vi "Initialize.vi"(8 "error in":errorcluster, 11 "Plugin in":refnum<class "RPM Plugin.lvclass">) -> (0 "error out":errorcluster, 3 "Plugin out":refnum<class "RPM Plugin.lvclass">)   [LabVIEW 2020, in "RPM Plugin.lvlib" / "RPM Plugin.lvclass"]
uses:
  RPM Plugin.lvclass
  C:/Program Files/National Instruments/LabVIEW 2020/vi.lib/FlexLogger/SDK/PluginSDK.lvlibp/PEFClasses/SDK/Plugin/Plugin.lvclass
  <vilib>/FlexLogger/SDK/PluginSDK.lvlibp/PEFClasses/SDK/Processing Element/Timing Parameters.ctl
  <vilib>/FlexLogger/SDK/PluginSDK.lvlibp/PEFClasses/SDK/Processing Element/Timing Method.ctl
  <vilib>/FlexLogger/SDK/PluginSDK.lvlibp/PEFClasses/SDK/Producer Channel/Producer Channel.lvclass
  C:/Program Files/National Instruments/LabVIEW 2020/vi.lib/FlexLogger/SDK/PluginSDK.lvlibp/PEFClasses/SDK/Channel/Channel.lvclass
  <vilib>/FlexLogger/SDK/PluginSDK.lvlibp/PEFClasses/SDK/Plugin/ParameterAccess/Write String.vi
  <vilib>/FlexLogger/SDK/PluginSDK.lvlibp/PEFClasses/SDK/Plugin/ParameterAccess/Write DBL.vi
  <vilib>/FlexLogger/SDK/PluginSDK.lvlibp/PEFClasses/SDK/Producer Channel/Create Producer Channel.vi
  <vilib>/FlexLogger/SDK/PluginSDK.lvlibp/PEFClasses/SDK/Channel/ParameterAccess/Write DBL.vi
  <vilib>/FlexLogger/SDK/PluginSDK.lvlibp/PEFClasses/SDK/Plugin/Plugin.lvclass
  <vilib>/FlexLogger/SDK/PluginSDK.lvlibp/PEFClasses/SDK/Channel/Channel.lvclass
  <vilib>/FlexLogger/SDK/PluginSDK.lvlibp
  <vilib>/FlexLogger/SDK/PluginSDK.lvlibp/PEFClasses/SDK/Processing Element/Processing Element.lvclass
  C:/Program Files/National Instruments/LabVIEW 2020/vi.lib/FlexLogger/SDK/PluginSDK.lvlibp/PEFClasses/SDK/Processing Element/Processing Element.lvclass
  D:/AE/Transportation/Schwing Stetter/RPM Plugin/RPM Plugin/RPM Plugin.lvclass
  C:/Program Files/National Instruments/LabVIEW 2020/vi.lib/FlexLogger/SDK/PluginSDK.lvlibp/PEFClasses/SDK/Producer Channel/Producer Channel.lvclass
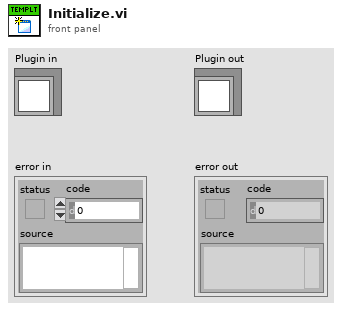
[diagram p1: front panel]
types:
  T1 = typedef "PluginSDK.lvlibp/Processing Element.lvclass/Timing Parameters.ctl" = cluster{"Timing Method":T2, "Timing Period (ms)":i32}
  T2 = typedef "PluginSDK.lvlibp/Processing Element.lvclass/Timing Method.ctl" = enum16{"Periodic", "Immediate", "On Data Ready", "Triggered"}
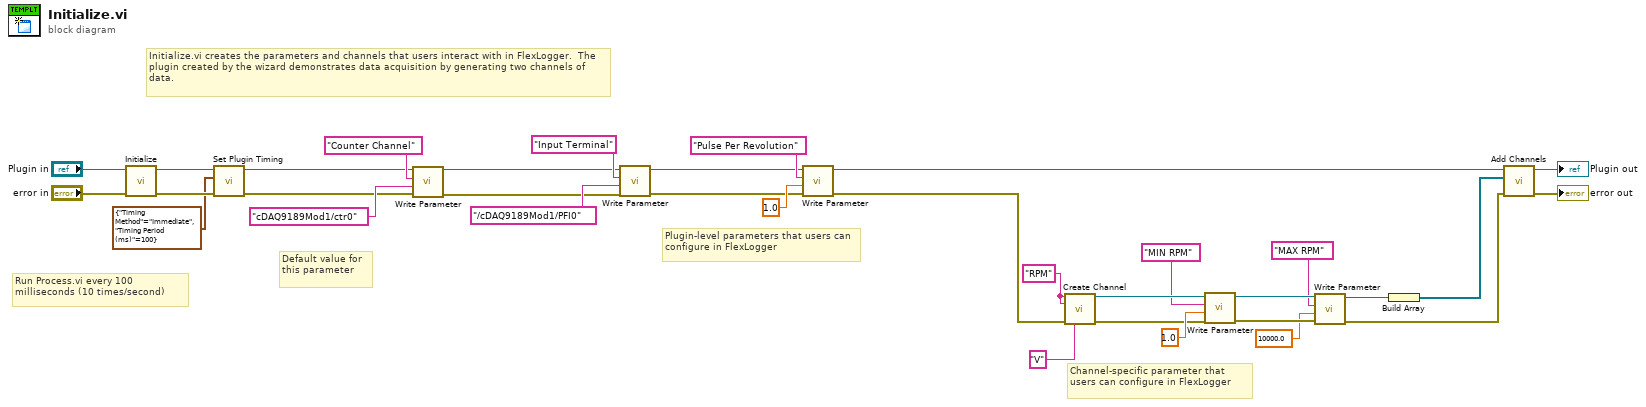
[diagram p0: block diagram]
diagram:
  w8 = "RPM" ("Unique Channel Identifier")
  # "Channel-specific parameter that users can configure in FlexLogger"
  # "Default value for this parameter"
  # "Plugin-level parameters that users can configure in FlexLogger"
  # "Run Process.vi every 100 milliseconds (10 times/second)"
  # "Initialize.vi creates the parameters and channels that users interact with in FlexLogger.  The plugin created by the wizard demonstrates data acquisition by generating two channels of data."
  n1 = call-parent "Initialize.vi"("error in (no error)"="error in", "Plugin in"="Plugin in") -> ("error out"=w24:errorcluster, "Plugin out"=w22:refnum<class "RPM Plugin.lvclass">)  [unwired: 8 in]
  n2 = call <vilib>:"Set Plugin Timing.vi"("error in (no error)"=w24, "Timing Parameters"=T1 {"Timing Method"=enum."Immediate", "Timing Period (ms)"=100}, "Plugin in"=w22) -> ("error out"=w20:errorcluster, "Plugin out"=w21:refnum<class "RPM Plugin.lvclass">)  [unwired: 7 in]
  n3 = call-poly <vilib>:"Write Parameter.vi"("error in (no error)"=w20, "Value"="cDAQ9189Mod1/ctr0", "Name"="Counter Channel", "Plugin in"=w21) -> ("error out"=w17:errorcluster, "Plugin out"=w14:refnum<class "RPM Plugin.lvclass">)  [unwired: 6 in]
  n4 = call-poly <vilib>:"Write Parameter.vi"("error in (no error)"=w17, "Value"="/cDAQ9189Mod1/PFI0", "Name"="Input Terminal", "Plugin in"=w14) -> ("error out"=w16:errorcluster, "Plugin out"=w15:refnum<class "RPM Plugin.lvclass">)  [unwired: 6 in]
  n5 = call-poly <vilib>:"Write Parameter.vi"("error in (no error)"=w16, "Value"=1.0, "Name"="Pulse Per Revolution", "Plugin in"=w15) -> ("error out"=w26:errorcluster, "Plugin out"=w30:refnum<class "RPM Plugin.lvclass">)  [unwired: 6 in]
  n6 = call-poly <vilib>:"Create Channel.vi"("Unique Channel Identifier"=w8, "Default Channel Name"=w8, "error in (no error)"=w26, "Unit"="V") -> ("Producer Channel"=w13:refnum<class "Producer Channel.lvclass">, "error out"=w9:errorcluster)  [unwired: 10 in]
  n7 = call-poly <vilib>:"Write Parameter.vi"("error in (no error)"=w9, "Value"=1.0, "Name"="MIN RPM", "Channel in"=w13) -> ("error out"=w7:errorcluster, "Channel out"=w5:refnum<class "Producer Channel.lvclass">)  [unwired: 6 in]
  n8 = call-poly <vilib>:"Write Parameter.vi"("error in (no error)"=w7, "Value"=10000.0, "Name"="MAX RPM", "Channel in"=w5) -> ("error out"=w6:errorcluster, "Channel out"=w2:refnum<class "Producer Channel.lvclass">)  [unwired: 6 in]
  n9 = Build Array(w2) -> (w1:refnum<class "Producer Channel.lvclass">[])
  n10 = call <vilib>:"Add Channels.vi"("error in (no error)"=w6, "Channels"=w1, "Plugin in"=w30) -> ("error out"=→"error out":errorcluster, "Plugin out"=→"Plugin out":refnum<class "RPM Plugin.lvclass">)  [unwired: 7 in]
